vi "Accelerometer control.vi"(4 "Enum":T1=enum."Run") -> (1 "Accelerations":cluster{"X Axis":dbl, "Y Axis":dbl})   [LabVIEW 2014]
uses:
  TypeDefs/SRE Enum.ctl
  <vilib>/addons/control/pid/pid.llb/PID Control Input Filter (DBL).vi
  <vilib>/Rock Robotics/WPI/Accelerometer/InternalAccelerometer/WPI_AccelerometerInternalOpen.vi
  <vilib>/addons/control/pid/NI_PID_pid.lvlib
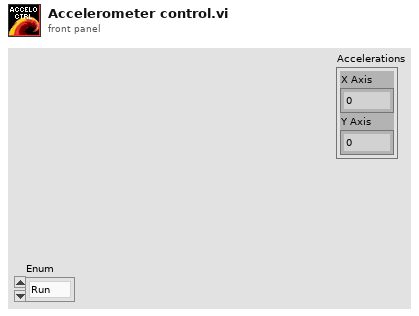
[diagram p1: front panel]
types:
  T1 = typedef "SRE Enum.ctl" = enum16{"Start", "Run", "End"}
  T2 = cluster{"X-Axis":dbl, "Y-Axis":dbl, "Z-Axis":dbl}
  T3 = typedef "WPI_AccelerometerDevRef.ctl" = cluster{"DevStatus":errorcluster, "Controller":T4, "Scaling":T5, "Analog Channels":T6, "I2C Bus":T8, "SPI Bus":T9, "Accel Range":T10, "ADXL345 Axes":T11, "Handle":i32, "Device Address":u8, "Accel Type":enum16{"Analog", "ADXL345 I2C", "ADXL345 SPI", "Internal"}}
  T4 = typedef "FPGA_TypedefAnalogModule.ctl" = enum16{"Controller 1"}
  T5 = typedef "WPI_AccelerometerScaling.ctl" = cluster{"Gain (VoltsPerG)":dbl, "Center Voltage":dbl}
  T6 = typedef "WPI_AccelerometerAnalogChannels.ctl" = cluster{"X-Axis":T7, "Y-Axis":T7, "Z-Axis":T7}
  T7 = typedef "FPGA_AIChannel.ctl" = enum8{"AI 0", "AI 1", "AI 2", "AI 3", "AI MXP 0", "AI MXP 1", "AI MXP 2", "AI MXP 3", "Invalid"}
  T8 = typedef "i2c_bus.ctl" = enum16{"I2C On-Board", "I2C MXP", "Invalid"}
  T9 = typedef "spi_bus.ctl" = enum16{"SPI On-Board, CS0", "SPI On-Board, CS1", "SPI On-Board, CS2", "SPI On-Board, CS3", "SPI MXP", "Invalid"}
  T10 = typedef "ADXL345 Range.ctl" = u8
  T11 = typedef "WPI_AccelerometerADXL345 Axes.ctl" = cluster{"X-Axis":bool, "Y-Axis":bool, "Z-Axis":bool}
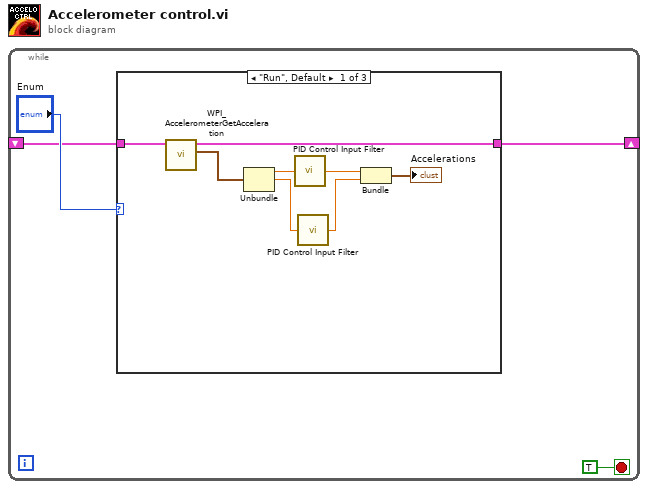
[diagram p0: block diagram]
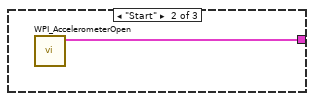
[diagram p2: hidden frame]
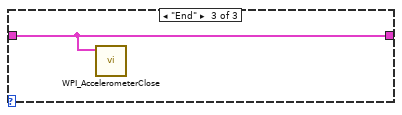
[diagram p3: hidden frame]
diagram:
  n1 = while {
    shift-right: [w3] -> _
    shift-left: _ -> [w2]
    stop <- TRUE stop-if-true
    n2 = case shown="\"Run\", Default" "Enum" {
      tunnel: [w11 w13 w14] -> w3
      tunnel: w2 -> [w12 _ w14]
      frame "Run", Default {
        n3 = call <vilib>:"WPI_AccelerometerGetAcceleration.vi"("AccelerometerDevRef"=w12) -> ("Accelerations"=w10:T2, "AccelerometerDevRef"=w11:T3)  [unwired: 8 in, 1 out]
        n4 = Unbundle(w10) -> ("X-Axis"=w9:dbl, "Y-Axis"=w8:dbl)  [unwired: 1 out]
        n5 = call-poly <vilib>:"PID Control Input Filter.vi"("input"=w9) -> ("output"=w7:dbl)  [unwired: 4 in]
        n6 = call-poly <vilib>:"PID Control Input Filter.vi"("input"=w8) -> ("output"=w6:dbl)  [unwired: 4 in]
        n7 = Bundle("output"=w7, "output"=w6) -> (→"Accelerations":cluster{"output":dbl, "output":dbl})  [unwired: 1 in]
      }
      frame "Start" {
        n8 = call-poly <vilib>:"WPI_AccelerometerOpen.vi"() -> ("AccelerometerDevRef"=w13:T3)  [unwired: 10 in, 1 out]
      }
      frame "End" {
        n9 = call <vilib>:"WPI_AccelerometerClose.vi"("AccelerometerDevRef"=w14) -> ()  [unwired: 10 in, 1 out]
      }
    }
  }
